vi "Set Test File Version.vi"(7 "Unique ID":string, 8 "error in (no error)":errorcluster, 10 "Test File Version":string, 11 "Test Executive Ref":refnum<data-value>) -> (0 "error out":errorcluster, 3 "Test Executive Ref out":refnum<data-value>)   [LabVIEW 2017, in "Test Executive.lvlib" / "TestExecutive Ref.lvclass"]
uses:
  <vilib>/gpm_packages/@cs/test-executive/Source/Test Executive/TestExecutive Ref/TestExecutive Ref.lvclass
  <vilib>/gpm_packages/@cs/test-executive/Source/Test Executive/ITestExecutive/ITest Executive.lvclass
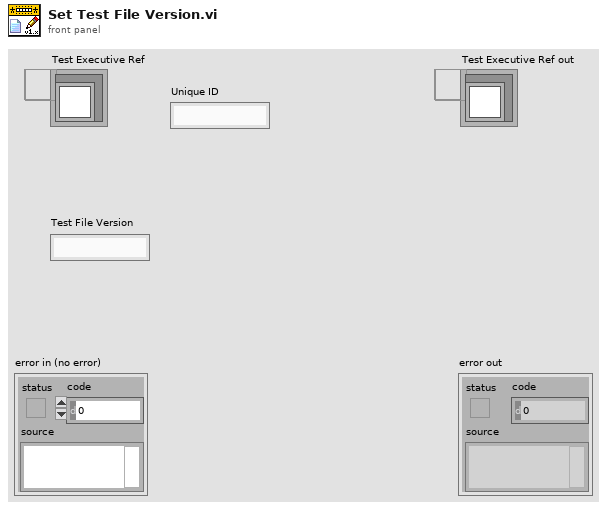
[diagram p1: front panel]
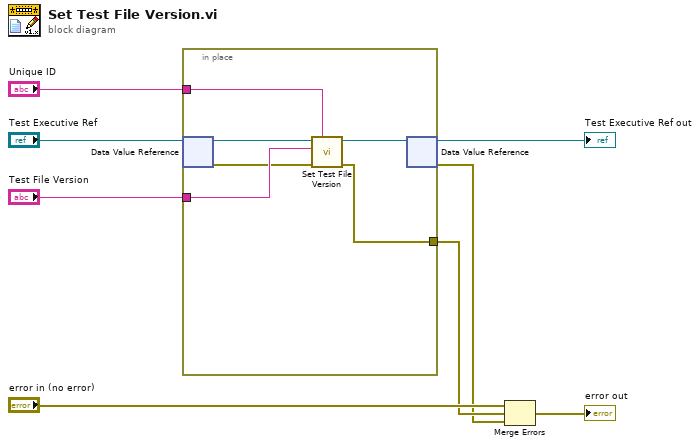
[diagram p0: block diagram]
diagram:
  n1 = in-place {
    in-place-border: "Unique ID" -> [w11]
    in-place-border: "Test File Version" -> [w12]
    in-place-border: [w9] -> w3
    n2 = in-place-dvr #1("Test Executive Ref") -> (w14:refnum<class "ITest Executive.lvclass">, w10:errorcluster)
    n3 = call-dynamic "Set Test File Version.vi"("Unique ID"=w11, "error in (no error)"=w10, "Test File Version"=w12, "ITest Executive in"=w14) -> ("error out"=w9:errorcluster, "ITest Executive out"=w13:refnum<class "ITest Executive.lvclass">)  [unwired: 6 in]
    n4 = in-place-dvr #1(w13) -> (→"Test Executive Ref out":refnum<data-value>, w2:errorcluster)
  }
  n5 = Merge Errors("error in (no error)", w3, w2) -> (→"error out":errorcluster)
